vi "Pre Launch Init.vi"(11 "Tiff Writer in":refnum<class "Tiff Writer.lvclass">) -> (0 "error out":errorcluster, 3 "Tiff Writer out":refnum<class "Tiff Writer.lvclass">)   [LabVIEW 2015]
doc: "(<B>Filename</B>: Actor Framework.lvlib:Actor.lvclass:Pre Launch Init.vi)\n\nDefines behavior that occurs after the Launch Nested Actor method is invoked but before the actor's Actor Core method begins running.\n\nBy default, this method does nothing. A descendant class may override it to define behavior."
uses:
  BinaryTIFF/Classes/TIFF/TIFF.lvclass
  Tiff Writer.lvclass
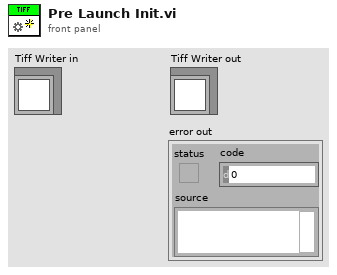
[diagram p1: front panel]
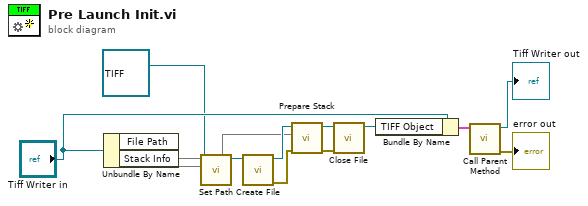
[diagram p0: block diagram]
diagram:
  n1 = Unbundle By Name("Tiff Writer in") -> ("File Path"=w11, "Stack Info"=w7)
  n2 = call-dynamic "Set Path.vi"("File Path"=w11, "TIFF in"=refnum<class "TIFF.lvclass"> refnum) -> ("TIFF out"=w10:refnum<class "TIFF.lvclass">)  [unwired: 8 in, 1 out]
  n3 = call-dynamic "Create File.vi"("TIFF in"=w10) -> ("error out"=w8:errorcluster, "TIFF out"=w9:refnum<class "TIFF.lvclass">)  [unwired: 9 in]
  n4 = call-dynamic "Prepare Stack.vi"("error in (no error)"=w8, "Stack Info"=w7, "TIFF in"=w9) -> ("error out"=w5:errorcluster, "TIFF out"=w6:refnum<class "TIFF.lvclass">)  [unwired: 7 in]
  n5 = call-dynamic "Close File.vi"("error in (no error)"=w5, "TIFF in"=w6) -> ("TIFF out"=w4:refnum<class "TIFF.lvclass">)  [unwired: 8 in, 1 out]
  n6 = Bundle By Name(cluster="Tiff Writer in", "TIFF Object"=w4) -> (w2:cluster{})
  n7 = call-parent "Call Parent Method"("Actor in"=w2) -> ("error out"=→"error out":errorcluster, "Actor out"=→"Tiff Writer out":refnum<class "Tiff Writer.lvclass">)  [unwired: 9 in]
